vi "list_files.vi"() -> ()   [LabVIEW 2021]
panel:
  out "selected item":string
  in  "stop":bool
  in  "Listbox":i32(listbox)
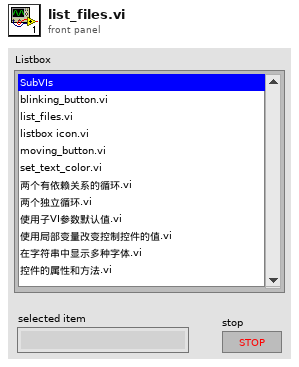
[diagram p1: front panel]
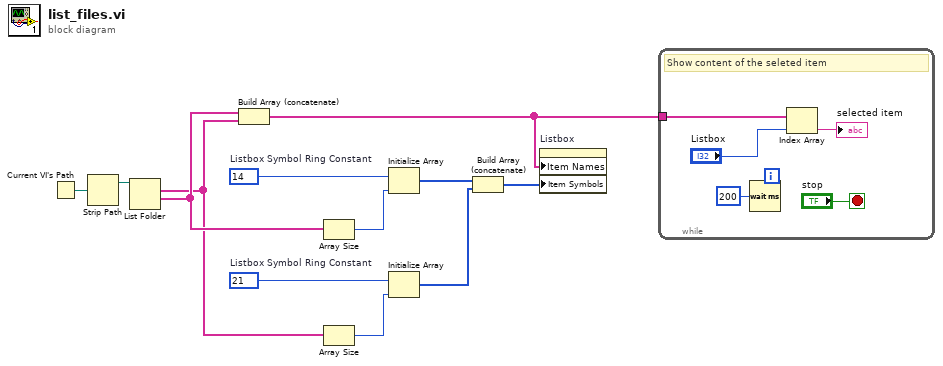
[diagram p0: block diagram]
diagram:
  w6 = 21  # Listbox Symbol Ring Constant
  w10 = 14  # Listbox Symbol Ring Constant
  n1 = Current VI's Path() -> (path=w12:path)
  n2 = Strip Path(path=w12) -> (stripped path=w11:path)  [unwired: 1 out]
  n3 = List Folder(path=w11) -> (filenames=w5:string[], folder names=w9:string[])  [unwired: 3 in, 2 out]
  n4 = Build Array (concatenate) "Build Array"(w9, w5) -> (w1:string[])
  n5 = Array Size(array=w9) -> (size(s)=w8:i32)
  n6 = Array Size(array=w5) -> (size(s)=w7:i32)
  n7 = Initialize Array "Initialize Array"(w10, w8) -> (w4:i32[])
  n8 = Initialize Array "Initialize Array"(w6, w7) -> (w3:i32[])
  n9 = Build Array (concatenate) "Build Array"(w4, w3) -> (w2:i32[])
  n10 = property on="Listbox" class="LstBox (strict)"("Item Names"=w1, "Item Symbols"=w2) -> ()  [unwired: 2 in, 2 out]
  n11 = while {
    tunnel: w1 -> [w16]
    stop <- "stop" stop-if-true
    # "Show content of the seleted item"
    n12 = Wait (ms)(milliseconds to wait=u32 200) -> ()  [unwired: 1 out]
    n13 = Index Array "Index Array"(array=w16, index="Listbox") -> (element=→"selected item":string)
  }
